vi "Always Positive.vi"(0 "Input":i32=-2) -> (6 "Output":i32=-2)   [LabVIEW 2014]
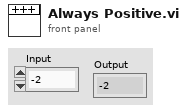
[diagram p1: front panel]
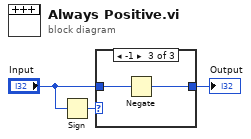
[diagram p0: block diagram]
diagram:
  n1 = Sign(1:"Input") -> (0:w2:i32)
  n2 = case shown="-1" w2 {
    tunnel: "Input" -> [w4 w5 w7]
    tunnel: [w4 w5 w6] -> w1
    frame 0, Default {
    }
    frame 1 {
    }
    frame -1 {
      n3 = Negate(x=w7) -> (-x=w6:i32)
    }
  }
  "Output" <- w1
